vi "ConvertToHandCount.vi"(1 "AddtionalTile":u16(ring)=36, 2 "Hand":u16[](array[ring])) -> (0 "HandCount":u16[](array[numeric]))   [LabVIEW 2025]
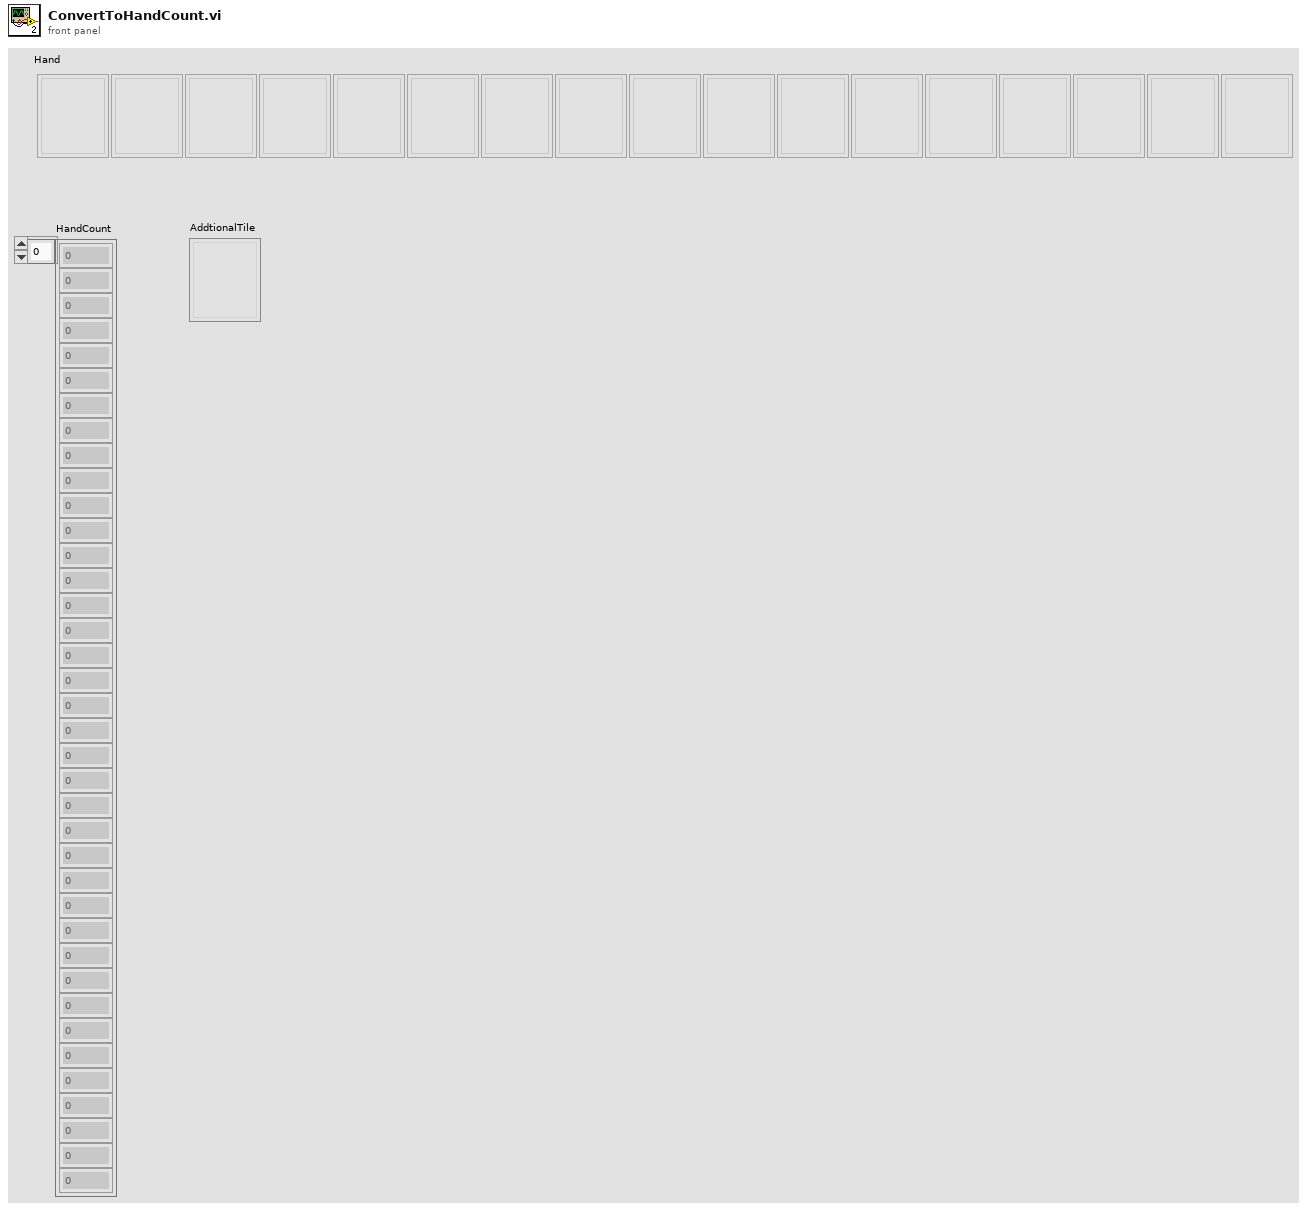
[diagram p1: front panel]
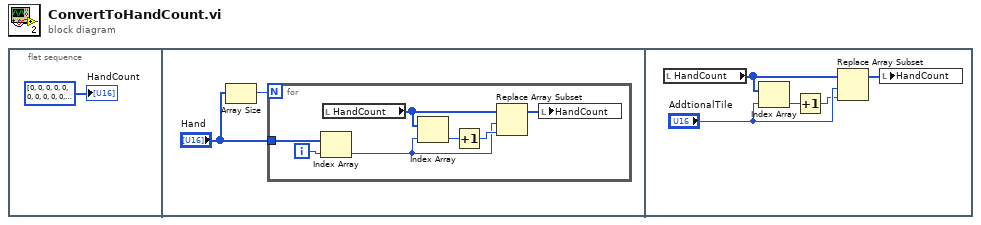
[diagram p0: block diagram]
diagram:
  n1 = flat-sequence {
    frame #0 {
      "HandCount" <- i32[] [0, 0, 0, 0, 0, 0, 0, 0, 0, 0, 0, 0, 0, 0, 0, 0, 0, 0, 0, 0, 0, 0, 0, 0, 0, 0, 0, 0, 0, 0, 0, 0, 0, 0, 0, 0, 0, 0]
    }
    frame #1 {
      n2 = Array Size(array="Hand") -> (size(s)=w3:i32)
      n3 = for {
        N: w3 -> [_]
        tunnel: "Hand" -> [w10]
        i -> [w9]
        n4 = Index Array(array=w10, index=w9) -> (element=w5:u16)
        n5 = local read "HandCount"() -> (w6:u16[])
        n6 = Index Array(array=w6, index=w5) -> (element=w7:u16)
        n7 = Increment(x=w7) -> (x+1=w8:u16)
        n8 = Replace Array Subset(array=w6, new element=w8, index=w5) -> (w4:u16[])
        n9 = local write "HandCount"(w4) -> ()
      }
    }
    frame #2 {
      n10 = local read "HandCount"() -> (w15:u16[])
      n11 = Index Array(array=w15, index="AddtionalTile") -> (element=w12:u16)
      n12 = Increment(x=w12) -> (x+1=w13:u16)
      n13 = Replace Array Subset(array=w15, new element=w13, index="AddtionalTile") -> (w11:u16[])
      n14 = local write "HandCount"(w11) -> ()
    }
  }
